vi "TwoCameraDisplayPanel.vi"() -> ()   [LabVIEW 2013]
uses:
  MvLVLib/MvCameraControl.lvlib
  MvLVLib/VIs/CreateGigEHandle.vi
  MvLVLib/VIs/CreateU3VHandle.vi
  <vilib>/picture/picture.llb/imagedata.ctl
panel:
  out "GenTLDeviceArray":T1(array[cluster])
  in  "image data 2":T2 caption="图像数据"
  in  "Rectangle 2":T3
  out "pFrameInfoEx out 2":T4
  in  "pConvertInfo In 2":T5
  out "nWidth 2":u32
  out "nHeight 2":u32
  out "PayloadSize 2":u32
  out "PixelFormat 2":u32
  out "handle out 2":u64
  in  "handle 2":u64
  out "Picture 2":picture
  in  "Device List 2":u16(ring)
  out "U3VDeviceArray":T6(array[cluster])
  out "GigEDeviceArray":T7(array[cluster])
  in  "pConvertInfo In":T5
  out "PixelFormat":u32
  out "handle out":u64
  in  "handle":u64
  in  "Rectangle":T3
  in  "image data":T2 caption="图像数据"
  out "Picture":picture
  out "PayloadSize":u32
  out "pFrameInfoEx out":T4
  out "nHeight":u32
  out "nWidth":u32
  out "Acquisision Flag":bool
  in  "Trigger Mode":bool
  in  "Continuous":bool
  out "打开标志":bool
  in  "stop":bool
  in  "Trigger Once":bool
  in  "Stop":bool
  in  "Start":bool
  in  "Open Device":bool
  in  "Close Device":bool
  in  "error in (no error) 2":errorcluster caption="错误输入（无错误）"
  in  "Refresh Devices":bool
  in  "Device List":u16(ring)
  # "Initialize"
  # "Acquisition"
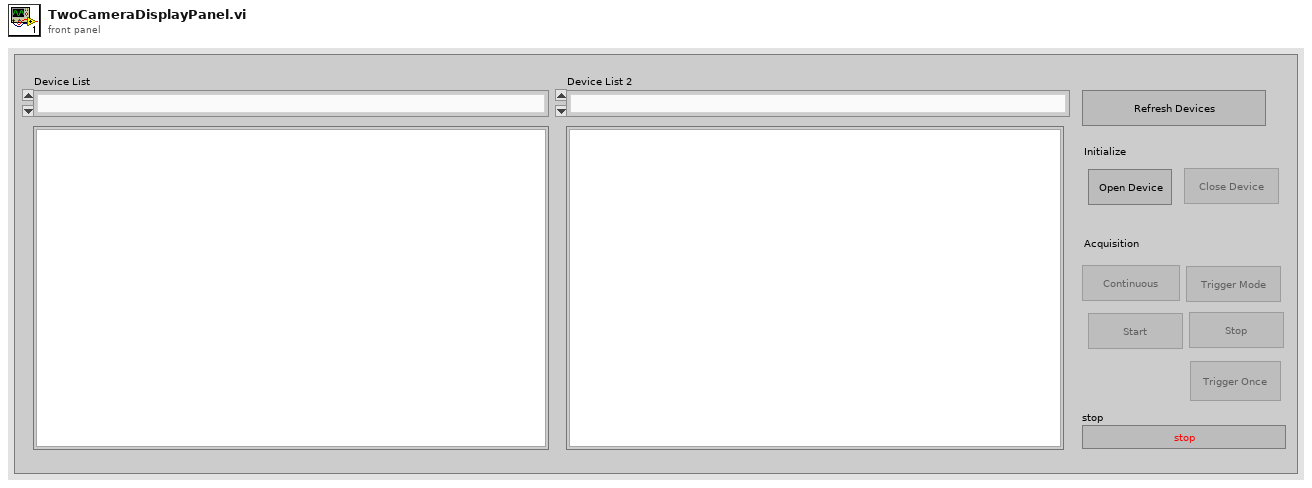
[diagram p1: front panel]
types:
  T1 = cluster{"nMajorVer":u16, "nMinorVer":u16, "nMacAddrHigh":u32, "nMacAddrLow":u32, "nTLayerType":u32, "nReserved0":u32, "nReserved1":u32, "nReserved2":u32, "nReserved3":u32, "chInterfaceID":string, "chVendorName":string, "chModelName":string, "chManufacturerInfo":string, "chDeviceVersion":string, "chSerialNumber":string, "chUserDefinedName":string, "chDeviceID":string, "nRes0":u32, "nRes1":u32, "nRes2":u32, "nRes3":u32, "nRes4":u32, "nRes5":u32, "nRes6":u32}[]
  T2 = typedef "imagedata.ctl" = cluster{"image type":i32, "image depth":i32, "image":u8[], "mask":u8[], "colors":u32[], "Rectangle":cluster{"left":i16, "top":i16, "right":i16, "bottom":i16}}
  T3 = cluster{"left":i16, "top":i16, "right":i16, "bottom":i16}
  T4 = cluster{"nWidth":u16, "nHeight":u16, "enPixelType":i32, "nFrameNum":u32, "nDevTimeStampHigh":u32, "nDevTimeStampLow":u32, "nReserved0":u32, "nHostTimeStamp":i64, "nFrameLen":u32, "nSecondCount]":u32, "nCycleCount":u32, "nCycleOffset":u32, "fGain":u32, "fExposureTime":u32, "nAverageBrightness":u32, "nRed":u32, "nGreen":u32, "nBlue":u32, "nFrameCounter":u32, "nTriggerIndex":u32, "nInput":u32, "nOutput":u32, "nOffsetX":u32, "nOffsetY":u32, "nReserved[0]":u32, "nReserved[1]":u32, "nReserved[2]":u32, "nReserved[3]":u32, "nReserved[4]":u32, "nReserved[5]":u32, "nReserved[6]":u32, "nReserved[7]":u32, "nReserved[8]":u32, "nReserved[9]":u32, "nReserved[10]":u32, "nReserved[11]":u32, "nReserved[12]":u32, "nReserved[13]":u32, "nReserved[14] 10":u32, "nReserved[15] 11":u32, "nReserved[16] 12":u32, "nReserved[17] 13":u32, "nReserved[18] 14":u32, "nReserved[19] 15":u32, "nReserved[20] 16":u32, "nReserved[21] 17":u32, "nReserved[22] 18":u32, "nReserved[23] 19":u32, "nReserved[24] 20":u32, "nReserved[25] 21":u32, "nReserved[26] 22":u32, "nReserved[27] 23":u32, "nReserved[28] 24":u32, "nReserved[29] 25":u32, "nReserved[30] 26":u32, "nReserved[31] 27":u32, "nReserved[32] 28":u32, "nReserved[33] 29":u32, "nReserved[34] 30":u32, "nReserved[35] 31":u32, "nReserved[36] 32":u32, "nReserved[37] 33":u32, "nReserved[38] 34":u32, "nReserved[39] 35":u32, "nReserved[40] 36":u32}
  T5 = cluster{"nWidth":u16, "nHeight":u16, "enSrcPixelType":u32, "nSrcDataLen":u32, "enDstPixelType":u32, "nDstLen":u32, "nDstBufferSize":u32, "nRes0":u32, "nRes1":u32, "nRes2":u32, "nRes3":u32}
  T6 = cluster{"nMajorVer":u16, "nMinorVer":u16, "nMacAddrHigh":u32, "nMacAddrLow":u32, "nTLayerType":u32, "nReserved0":u32, "nReserved1":u32, "nReserved2":u32, "nReserved3":u32, "CrtlInEndPoint":u8, "CrtlOutEndPoint":u8, "StreamEndPoint":u8, "EventEndPoint":u8, "idVendor":u16, "idProduct":u16, "nDeviceNumber":u32, "chDeviceGUID":string, "chVendorName":string, "chModelName":string, "chFamilyName":string, "chDeviceVersion":string, "chManufacturerName":string, "chSerialNumber":string, "chUserDefinedName":string, "nbcdUSB":u32, "nDeviceAddress":u32, "nRes0":u32, "nRes1":u32, "nResAlign":u32}[]
  T7 = cluster{"nMajorVer":u16, "nMinorVer":u16, "nMacAddrHigh":u32, "nMacAddrLow":u32, "nTLayerType":u32, "nReserved0":u32, "nReserved1":u32, "nReserved2":u32, "nReserved3":u32, "nIpCfgOption":u32, "nIpCfgCurrent":u32, "nCurrentIp":u32, "nCurrentSubNetMask":u32, "nDefaultGateWay":u32, "chManualfacturerName":string, "chModelName":string, "chDeviceVersion":string, "chManufacturerSpecificInfo":string, "chSerialNumber":string, "chUserDefinedName":string, "nNetExport":u32, "nRes0":u32, "nRes1":u32, "nRes2":u32, "nRes3":u32}[]
  T8 = enum8{"Enabled", "Disabled", "Disabled and Grayed Out"}
  T9 = cluster{"nCurValue":u32, "nMax":u32, "nMin":u32, "nInc":u32, "nReserved[0]":u32, "nReserved[1]":u32, "nReserved[2]":u32, "nReserved[3]":u32}
  T10 = cluster{"nCurValue":u32, "nSupportedNum":u32, "nSupportValue":u32[], "nReserved[0]":u32, "nReserved[1]":u32, "nReserved[2]":u32, "nReserved[3]":u32}
  T11 = cluster{"nMajorVer":u16, "nMinorVer":u16, "nMacAddrHigh":u32, "nMacAddrLow":u32, "nTLayerType":u32, "nReserved0":u32, "nReserved1":u32, "nReserved2":u32, "nReserved3":u32, "nIpCfgOption":u32, "nIpCfgCurrent":u32, "nCurrentIp":u32, "nCurrentSubNetMask":u32, "nDefaultGateWay":u32, "chManualfacturerName":string, "chModelName":string, "chDeviceVersion":string, "chManufacturerSpecificInfo":string, "chSerialNumber":string, "chUserDefinedName":string, "nNetExport":u32, "nRes0":u32, "nRes1":u32, "nRes2":u32, "nRes3":u32}
  T12 = cluster{"nMajorVer":u16, "nMinorVer":u16, "nMacAddrHigh":u32, "nMacAddrLow":u32, "nTLayerType":u32, "nReserved0":u32, "nReserved1":u32, "nReserved2":u32, "nReserved3":u32, "CrtlInEndPoint":u8, "CrtlOutEndPoint":u8, "StreamEndPoint":u8, "EventEndPoint":u8, "idVendor":u16, "idProduct":u16, "nDeviceNumber":u32, "chDeviceGUID":string, "chVendorName":string, "chModelName":string, "chFamilyName":string, "chDeviceVersion":string, "chManufacturerName":string, "chSerialNumber":string, "chUserDefinedName":string, "nbcdUSB":u32, "nDeviceAddress":u32, "nRes0":u32, "nRes1":u32, "nResAlign":u32}
  T13 = cluster{"nMajorVer":u16, "nMinorVer":u16, "nMacAddrHigh":u32, "nMacAddrLow":u32, "nTLayerType":u32, "nReserved0":u32, "nReserved1":u32, "nReserved2":u32, "nReserved3":u32, "chInterfaceID":string, "chVendorName":string, "chModelName":string, "chManufacturerInfo":string, "chDeviceVersion":string, "chSerialNumber":string, "chUserDefinedName":string, "chDeviceID":string, "nRes0":u32, "nRes1":u32, "nRes2":u32, "nRes3":u32, "nRes4":u32, "nRes5":u32, "nRes6":u32}
  T14 = cluster{"nWidth":u32, "nHeight":u32, "enSrcPixelType":u32, "nSrcDataLen":u32, "enDstPixelType":u32, "nDstLen":u32, "nDstBufferSize":u32, "nRes0":u32, "nRes1":u32, "nRes2":u32, "nRes3":u32}
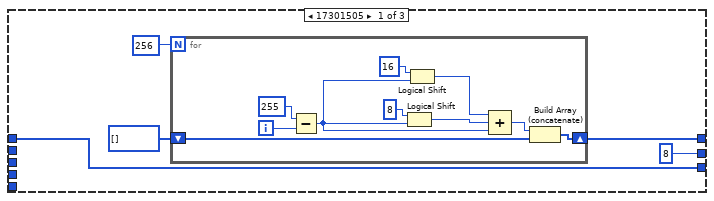
[diagram p9: hidden frame]
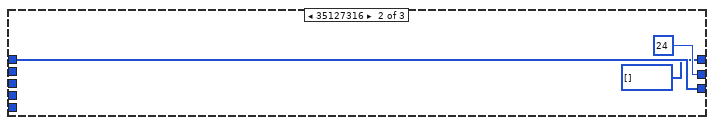
[diagram p10: hidden frame]
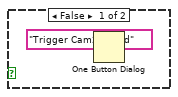
[diagram p12: hidden frame]
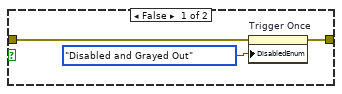
[diagram p17: hidden frame]
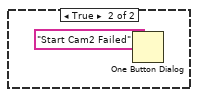
[diagram p18: hidden frame]
diagram:
  n1 = while {
    tunnel: ["stop"] -> w3
    shift-right: [w41] -> _
    shift-left: "handle" -> [_]
    tunnel: ["stop"] -> w1
    tunnel: [w10] -> _
    stop <- "stop" stop-if-true
    n2 = property on="handle out" class="DigNum (strict)"() -> ("Value"=w33:u64)  [unwired: 2 in, 2 out]
    n3 = property on="handle out" class="DigNum (strict)"() -> ("Value"=w39:u64)  [unwired: 2 in, 2 out]
    n4 = property on="handle out" class="DigNum (strict)"() -> ("Value"=w34:u64)  [unwired: 2 in, 2 out]
    n5 = property on="handle out" class="DigNum (strict)"() -> ("Value"=w35:u64)  [unwired: 2 in, 2 out]
    n6 = property on="handle out 2" class="DigNum (strict)"() -> ("Value"=w24:u64)  [unwired: 2 in, 2 out]
    n7 = property on="handle out" class="DigNum (strict)"() -> ("Value"=w38:u64)  [unwired: 2 in, 2 out]
    n8 = property on="handle out" class="DigNum (strict)"() -> ("Value"=w37:u64)  [unwired: 2 in, 2 out]
    n9 = property on="handle out 2" class="DigNum (strict)"() -> ("Value"=w18:u64)  [unwired: 2 in, 2 out]
    n10 = property on="handle out 2" class="DigNum (strict)"() -> ("Value"=w17:u64)  [unwired: 2 in, 2 out]
    n11 = case shown="True" "Trigger Mode" {
      tunnel: w34 -> [_ w401]
      frame False {
      }
      frame True {
        n12 = call "SetEnumValue.vi"("nValue"=u32 1, "strKey"="TriggerMode", "handle"=w401) -> ("error out"=w407:errorcluster)  [unwired: 6 in, 2 out]
        n13 = call "SetEnumValue.vi"("error in (no error)"=w407, "nValue"=u32 7, "strKey"="TriggerSource", "handle"=w401) -> ("error out"=w406:errorcluster)  [unwired: 5 in, 2 out]
        n14 = property on="Trigger Mode" class="Bool"(error in=w406, "DisabledEnum"=T8."Disabled and Grayed Out" ("禁用")) -> (error out=w405:errorcluster)  [unwired: 1 in, 1 out]
        n15 = property on="Continuous" class="Bool"(error in=w405, "DisabledEnum"=T8."Enabled" ("禁用")) -> (error out=w403:errorcluster)  [unwired: 1 in, 1 out]
        n16 = property on="Trigger Once" class="Bool"(error in=w403, "DisabledEnum"=T8."Enabled" ("禁用")) -> ()  [unwired: 1 in, 2 out]
      }
    }
    n17 = case shown="True" "Trigger Once" {
      tunnel: w38 -> [_ w416]
      frame False {
      }
      frame True {
        n18 = call "SetCommandValue.vi"("strValue"="TriggerSoftware", "handle"=w416) -> ("function return"=w414:i32)  [unwired: 7 in, 2 out]
        n19 = Equal To 0?(x=w414) -> (x = 0?=w413:bool)
        n20 = case shown="True" w413 {
          frame False {
            n21 = One Button Dialog(message="Trigger Cam1 Failed") -> ()  [unwired: 1 in, 1 out]
          }
          frame True {
            n22 = One Button Dialog(message="Trigger Can1 Success") -> ()  [unwired: 1 in, 1 out]
          }
        }
      }
    }
    n23 = case shown="True" "Stop" {
      tunnel: w37 -> [_ w391]
      frame False {
      }
      frame True {
        n24 = call "StopGrabbing.vi"("handle"=w391) -> ("error out"=w390:errorcluster)  [unwired: 8 in, 2 out]
        n25 = property on="Acquisision Flag" class="Bool (strict)"(error in=w390, "Value"=FALSE ("采集标志")) -> (error out=w385:errorcluster)  [unwired: 1 in, 1 out]
        n26 = property on="Start" class="Bool"(error in=w385, "DisabledEnum"=T8."Enabled" ("禁用")) -> (error out=w384:errorcluster)  [unwired: 1 in, 1 out]
        n27 = property on="Stop" class="Bool"(error in=w384, "DisabledEnum"=T8."Disabled and Grayed Out" ("禁用")) -> (error out=w383:errorcluster)  [unwired: 1 in, 1 out]
        n28 = property on="Trigger Once" class="Bool"(error in=w383, "DisabledEnum"=T8."Disabled and Grayed Out" ("禁用")) -> ()  [unwired: 1 in, 2 out]
      }
    }
    n29 = case shown="True" "Continuous" {
      tunnel: w33 -> [_ w392]
      frame False {
      }
      frame True {
        n30 = call "SetEnumValue.vi"("nValue"=u32 0, "strKey"="TriggerMode", "handle"=w392) -> ("error out"=w393:errorcluster)  [unwired: 6 in, 2 out]
        n31 = property on="Continuous" class="Bool"(error in=w393, "DisabledEnum"=T8."Disabled and Grayed Out" ("禁用")) -> (error out=w397:errorcluster)  [unwired: 1 in, 1 out]
        n32 = property on="Trigger Mode" class="Bool"(error in=w397, "DisabledEnum"=T8."Enabled" ("禁用")) -> (error out=w395:errorcluster)  [unwired: 1 in, 1 out]
        n33 = property on="Trigger Once" class="Bool"(error in=w395, "DisabledEnum"=T8."Disabled and Grayed Out" ("禁用")) -> ()  [unwired: 1 in, 2 out]
      }
    }
    n34 = case shown="True" "Stop" {
      tunnel: w18 -> [_ w147]
      frame False {
      }
      frame True {
        n35 = call "StopGrabbing.vi"("handle"=w147) -> ("error out"=w146:errorcluster)  [unwired: 8 in, 2 out]
        n36 = property on="Acquisision Flag" class="Bool (strict)"(error in=w146, "Value"=FALSE ("采集标志")) -> (error out=w141:errorcluster)  [unwired: 1 in, 1 out]
        n37 = property on="Start" class="Bool"(error in=w141, "DisabledEnum"=T8."Enabled" ("禁用")) -> (error out=w140:errorcluster)  [unwired: 1 in, 1 out]
        n38 = property on="Stop" class="Bool"(error in=w140, "DisabledEnum"=T8."Disabled and Grayed Out" ("禁用")) -> (error out=w139:errorcluster)  [unwired: 1 in, 1 out]
        n39 = property on="Trigger Once" class="Bool"(error in=w139, "DisabledEnum"=T8."Disabled and Grayed Out" ("禁用")) -> ()  [unwired: 1 in, 2 out]
      }
    }
    n40 = case shown="True" "Trigger Once" {
      tunnel: w17 -> [_ w136]
      frame False {
      }
      frame True {
        n41 = call "SetCommandValue.vi"("strValue"="TriggerSoftware", "handle"=w136) -> ("function return"=w134:i32)  [unwired: 7 in, 2 out]
        n42 = Equal To 0?(x=w134) -> (x = 0?=w133:bool)
        n43 = case shown="True" w133 {
          frame False {
            n44 = One Button Dialog(message="Trigger Cam2 Failed") -> ()  [unwired: 1 in, 1 out]
          }
          frame True {
            n45 = One Button Dialog(message="Trigger Cam2 Success") -> ()  [unwired: 1 in, 1 out]
          }
        }
      }
    }
    n46 = case shown="True" "Close Device" {
      tunnel: w39 -> [_ w462]
      frame False {
      }
      frame True {
        n47 = call "CloseDevice.vi"("handle"=w462) -> ("error out"=w464:errorcluster, "handle out"=w461:u64)  [unwired: 8 in, 1 out]
        n48 = call "DestroyHandle.vi"("error in (no error)"=w464, "handle"=w461) -> ("error out"=w463:errorcluster)  [unwired: 8 in, 1 out]
        n49 = property on="Open Device" class="Bool"(error in=w463, "DisabledEnum"=T8."Enabled" ("禁用")) -> (error out=w477:errorcluster)  [unwired: 1 in, 1 out]
        n50 = property on="Close Device" class="Bool"(error in=w477, "DisabledEnum"=T8."Disabled and Grayed Out" ("禁用")) -> (error out=w476:errorcluster)  [unwired: 1 in, 1 out]
        n51 = property on="Start" class="Bool"(error in=w476, "DisabledEnum"=T8."Disabled and Grayed Out" ("禁用")) -> (error out=w475:errorcluster)  [unwired: 1 in, 1 out]
        n52 = property on="Stop" class="Bool"(error in=w475, "DisabledEnum"=T8."Disabled and Grayed Out" ("禁用")) -> (error out=w474:errorcluster)  [unwired: 1 in, 1 out]
        n53 = property on="Trigger Once" class="Bool"(error in=w474, "DisabledEnum"=T8."Disabled and Grayed Out" ("禁用")) -> (error out=w471:errorcluster)  [unwired: 1 in, 1 out]
        n54 = property on="Continuous" class="Bool"(error in=w471, "DisabledEnum"=T8."Disabled and Grayed Out" ("禁用")) -> (error out=w469:errorcluster)  [unwired: 1 in, 1 out]
        n55 = property on="Trigger Mode" class="Bool"(error in=w469, "DisabledEnum"=T8."Disabled and Grayed Out" ("禁用")) -> (error out=w468:errorcluster)  [unwired: 1 in, 1 out]
        n56 = property on="打开标志" class="Bool (strict)"(error in=w468, "Value"=FALSE ("打开标志")) -> (error out=w466:errorcluster)  [unwired: 1 in, 1 out]
        n57 = property on="Acquisision Flag" class="Bool (strict)"(error in=w466, "Value"=FALSE ("采集标志")) -> ()  [unwired: 1 in, 2 out]
      }
    }
    n58 = case shown="True" "Refresh Devices" {
      tunnel: [w547 w556] -> w29
      tunnel: "error in (no error) 2" -> [w547 w555]
      frame False {
        n59 = property on="GigEDeviceArray" class="Arr (strict)" props=["Value"]() -> ()  [unwired: 2 in, 3 out]
        n60 = property on="U3VDeviceArray" class="Arr (strict)" props=["Value"]() -> ()  [unwired: 2 in, 3 out]
      }
      frame True {
        n61 = call "EnumDevicesEx2.vi"("nLayerType"=u32 965, "error in (no error)"=w555) -> ("GigEDeviceArray"=w552:T7, "U3VDeviceArray"=w550:T6, "GenTLDevice"=w549:T1, "error out"=w556:errorcluster)  [unwired: 8 in, 2 out]
        "GigEDeviceArray" <- w552
        "U3VDeviceArray" <- w550
        "GenTLDeviceArray" <- w549
        n62 = for {
          tunnel: w556 -> [_]
          tunnel: w552 -> [w583] mode=indexing
          tunnel: [w582] -> w554 mode=indexing
          n63 = Unbundle By Name(w583) -> ("chUserDefinedName"=w586:string)
          n64 = Unbundle By Name(w583) -> ("chSerialNumber"=w584:string)
          n65 = Unbundle By Name(w583) -> ("chModelName"=w585:string)
          n66 = call <vilib>:"Space Constant.vi"() -> ("String"=w589:string)
          n67 = Concatenate Strings("[GigE] " ("字符串"), w586, w589, w585, "(" ("字符串"), w584, ")" ("字符串")) -> (w582:string)
        }
        n68 = for {
          tunnel: w550 -> [w576] mode=indexing
          tunnel: [w573] -> w553 mode=indexing
          n69 = Unbundle By Name(w576) -> ("chUserDefinedName"=w580:string)
          n70 = Unbundle By Name(w576) -> ("chSerialNumber"=w575:string)
          n71 = Unbundle By Name(w576) -> ("chModelName"=w578:string)
          n72 = call <vilib>:"Space Constant.vi"() -> ("String"=w579:string)
          n73 = Concatenate Strings("[U3V] " ("字符串"), w580, w579, w578, "(" ("字符串"), w575, ")" ("字符串")) -> (w573:string)
        }
        n74 = for {
          tunnel: w549 -> [w564] mode=indexing
          tunnel: [w562] -> w548 mode=indexing
          n75 = Unbundle By Name(w564) -> ("nTLayerType"=w559:u32, "chUserDefinedName"=w567:string, "chModelName"=w561:string, "chSerialNumber"=w560:string)
          n76 = case shown="80" w559 {
            tunnel: ["[GenTL]" ("字符串") "[GenTL CML]" ("字符串") "[GenTL CXP]" ("字符串") "[GenTL XOF]" ("字符串")] -> w558
            frame Default {
            }
            frame 128 {
            }
            frame 256 {
            }
            frame 512 {
            }
          }
          n77 = call <vilib>:"Space Constant.vi"() -> ("String"=w566:string)
          n78 = Concatenate Strings(w558, w567, w566, w561, "(" ("字符串"), w560, ")" ("字符串")) -> (w562:string)
        }
        n79 = Build Array (concatenate)(w554, w553, w548) -> (w551:string[])
        n80 = property on="Device List" class="Ring (strict)"("Strings []"=w551) -> ()  [unwired: 2 in, 2 out]
        n81 = property on="Device List 2" class="Ring (strict)"("Strings []"=w551) -> ()  [unwired: 2 in, 2 out]
      }
    }
    n82 = case shown="True" "Start" {
      tunnel: w35 -> [_ w423]
      frame False {
      }
      frame True {
        n83 = call "GetIntValue.vi"("strKey"="PayloadSize", "handle"=w423) -> ("error out"=w429:errorcluster, "pIntValue out"=w425:T9, "handle out"=w421:u64)  [unwired: 6 in, 1 out]
        n84 = Unbundle By Name(w425) -> ("nCurValue"=→"PayloadSize":u32)
        n85 = call "GetEnumValue.vi"("error in (no error)"=w429, "strKey"="PixelFormat", "handle"=w421) -> ("error out"=w428:errorcluster, "pEnumValue out"=w430:T10, "handle out"=w420:u64)  [unwired: 5 in, 1 out]
        n86 = Unbundle By Name(w430) -> ("nCurValue"=→"PixelFormat":u32)
        n87 = call "StartGrabbing.vi"("error in (no error)"=w428, "handle"=w420) -> ("error out"=w427:errorcluster, "function return"=w433:i32, "handle out"=w419:u64)  [unwired: 7 in]
        n88 = Not Equal To 0?(x=w433) -> (x != 0?=w432:bool)
        n89 = case shown="True" w432 {
          tunnel: w423 -> [_ _]
          tunnel: w427 -> [w436 _]
          tunnel: w419 -> [w435 _]
          frame False {
            n90 = call "GetIntValue.vi"("error in (no error)"=w436, "strKey"="Width", "handle"=w435) -> ("error out"=w443:errorcluster, "pIntValue out"=w437:T9, "handle out"=w434:u64)  [unwired: 5 in, 1 out]
            n91 = Unbundle By Name(w437) -> ("nCurValue"=→"nWidth":u32)
            n92 = call "GetIntValue.vi"("error in (no error)"=w443, "strKey"="Height", "handle"=w434) -> ("error out"=w442:errorcluster, "pIntValue out"=w440:T9)  [unwired: 5 in, 2 out]
            n93 = Unbundle By Name(w440) -> ("nCurValue"=→"nHeight":u32)
            n94 = property on="Start" class="Bool"(error in=w442, "DisabledEnum"=T8."Disabled and Grayed Out" ("禁用")) -> (error out=w452:errorcluster)  [unwired: 1 in, 1 out]
            n95 = property on="Stop" class="Bool"(error in=w452, "DisabledEnum"=T8."Enabled" ("禁用")) -> (error out=w438:errorcluster)  [unwired: 1 in, 1 out]
            n96 = property on="Continuous" class="Bool"(error in=w438) -> (error out=w448:errorcluster, "DisabledEnum"=w449:T8)  [unwired: 1 in, 1 out]
            n97 = Equal To 0?(x=w449) -> (x = 0?=w450:bool)
            n98 = case shown="True" w450 {
              tunnel: w448 -> [w455 w458]
              tunnel: [w454 w457] -> w447
              frame False {
                n99 = property on="Trigger Once" class="Bool"(error in=w455, "DisabledEnum"=T8."Disabled and Grayed Out" ("禁用")) -> (error out=w454:errorcluster)  [unwired: 1 in, 1 out]
              }
              frame True {
                n100 = property on="Trigger Once" class="Bool"(error in=w458, "DisabledEnum"=T8."Enabled" ("禁用")) -> (error out=w457:errorcluster)  [unwired: 1 in, 1 out]
              }
            }
            n101 = property on="Acquisision Flag" class="Bool (strict)"(error in=w447, "Value"=TRUE ("采集标志")) -> ()  [unwired: 1 in, 2 out]
          }
          frame True {
            n102 = One Button Dialog(message="Start Cam1 Failed") -> ()  [unwired: 1 in, 1 out]
          }
        }
      }
    }
    n103 = case shown="True" "Start" {
      tunnel: w24 -> [_ w171]
      frame False {
      }
      frame True {
        n104 = call "GetIntValue.vi"("strKey"="PayloadSize", "handle"=w171) -> ("error out"=w177:errorcluster, "pIntValue out"=w173:T9, "handle out"=w169:u64)  [unwired: 6 in, 1 out]
        n105 = Unbundle By Name(w173) -> ("nCurValue"=→"PayloadSize 2":u32)
        n106 = call "GetEnumValue.vi"("error in (no error)"=w177, "strKey"="PixelFormat", "handle"=w169) -> ("error out"=w176:errorcluster, "pEnumValue out"=w178:T10, "handle out"=w168:u64)  [unwired: 5 in, 1 out]
        n107 = Unbundle By Name(w178) -> ("nCurValue"=→"PixelFormat 2":u32)
        n108 = call "StartGrabbing.vi"("error in (no error)"=w176, "handle"=w168) -> ("error out"=w175:errorcluster, "function return"=w181:i32, "handle out"=w167:u64)  [unwired: 7 in]
        n109 = Not Equal To 0?(x=w181) -> (x != 0?=w180:bool)
        n110 = case shown="False" w180 {
          tunnel: w171 -> [_ _]
          tunnel: w175 -> [w186 _]
          tunnel: w167 -> [w185 _]
          frame False {
            n111 = call "GetIntValue.vi"("error in (no error)"=w186, "strKey"="Width", "handle"=w185) -> ("error out"=w192:errorcluster, "pIntValue out"=w187:T9, "handle out"=w184:u64)  [unwired: 5 in, 1 out]
            n112 = Unbundle By Name(w187) -> ("nCurValue"=→"nWidth 2":u32)
            n113 = call "GetIntValue.vi"("error in (no error)"=w192, "strKey"="Height", "handle"=w184) -> ("error out"=w183:errorcluster, "pIntValue out"=w190:T9)  [unwired: 5 in, 2 out]
            n114 = Unbundle By Name(w190) -> ("nCurValue"=→"nHeight 2":u32)
            n115 = property on="Start" class="Bool"(error in=w183, "DisabledEnum"=T8."Disabled and Grayed Out" ("禁用")) -> ()  [unwired: 1 in, 2 out]
            n116 = property on="Stop" class="Bool"("DisabledEnum"=T8."Enabled" ("禁用")) -> (error out=w188:errorcluster)  [unwired: 2 in, 1 out]
            n117 = property on="Continuous" class="Bool"(error in=w188) -> (error out=w197:errorcluster, "DisabledEnum"=w198:T8)  [unwired: 1 in, 1 out]
            n118 = Equal To 0?(x=w198) -> (x = 0?=w199:bool)
            n119 = case shown="True" w199 {
              tunnel: w197 -> [w202 w205]
              tunnel: [w201 w204] -> w196
              frame False {
                n120 = property on="Trigger Once" class="Bool"(error in=w202, "DisabledEnum"=T8."Disabled and Grayed Out" ("禁用")) -> (error out=w201:errorcluster)  [unwired: 1 in, 1 out]
              }
              frame True {
                n121 = property on="Trigger Once" class="Bool"(error in=w205, "DisabledEnum"=T8."Enabled" ("禁用")) -> (error out=w204:errorcluster)  [unwired: 1 in, 1 out]
              }
            }
            n122 = property on="Acquisision Flag" class="Bool (strict)"(error in=w196, "Value"=TRUE ("采集标志")) -> ()  [unwired: 1 in, 2 out]
          }
          frame True {
            n123 = One Button Dialog(message="Start Cam2 Failed") -> ()  [unwired: 1 in, 1 out]
          }
        }
      }
    }
    n124 = property on="PayloadSize" class="DigNum (strict)"() -> ("Value"=w30:u32)  [unwired: 2 in, 2 out]
    n125 = property on="PayloadSize 2" class="DigNum (strict)"() -> ("Value"=w12:u32)  [unwired: 2 in, 2 out]
    n126 = property on="handle out" class="DigNum (strict)"() -> ("Value"=w36:u64)  [unwired: 2 in, 2 out]
    n127 = property on="Acquisision Flag" class="Bool (strict)"() -> ("Value"=w8:bool)  [unwired: 2 in, 2 out]
    n128 = property on="Acquisision Flag" class="Bool (strict)"() -> ("Value"=w9:bool)  [unwired: 2 in, 2 out]
    n129 = Initialize Array(u8 0 ("元素"), w30) -> (w31:u8[])
    n130 = property on="handle out 2" class="DigNum (strict)"() -> ("Value"=w15:u64)  [unwired: 2 in, 2 out]
    n131 = Initialize Array(u8 0 ("元素"), w12) -> (w13:u8[])
    n132 = property on="handle out 2" class="DigNum (strict)"() -> ("Value"=w20:u64)  [unwired: 2 in, 2 out]
    n133 = property on="handle out 2" class="DigNum (strict)"() -> ("Value"=w22:u64)  [unwired: 2 in, 2 out]
    n134 = property on="handle" class="DigNum (strict)"() -> ("Value"=w40:u64)  [unwired: 2 in, 2 out]
    n135 = case shown="True" "Open Device" {
      tunnel: [w482 w495] -> _
      tunnel: w40 -> [w482 w484]
      tunnel: w29 -> [_ w490]
      frame False {
      }
      frame True {
        n136 = property on="handle out" class="DigNum (strict)"() -> ("Value"=w492:u64)  [unwired: 2 in, 2 out]
        n137 = property on="Device List" class="Ring (strict)"() -> ("RingText.Text"=w488:string)  [unwired: 2 in, 2 out]
        n138 = call "DestroyHandle.vi"("error in (no error)"=w490, "handle"=w492) -> ("error out"=w491:errorcluster)  [unwired: 8 in, 1 out]
        n139 = call <vilib>:"Clear Errors.vi"("error in (no error)"=w491) -> ("error out"=w483:errorcluster)  [unwired: 5 in, 1 out]
        n140 = String Subset(string=w488, length (rest)=5 ("长度（剩余）")) -> (substring=w487:string)  [unwired: 1 in]
        n141 = case shown="\"[GenT\"" w487 {
          tunnel: [w504 w510 w522 w525] -> w486
          tunnel: [w503 w509 w521 w526] -> w485
          tunnel: w484 -> [_ _ _ w526]
          tunnel: w483 -> [_ _ _ w525]
          frame "[GigE" {
            n142 = local read "GigEDeviceArray"() -> (w502:T7)
            n143 = property on="Device List" class="Ring (strict)"() -> ("Value"=w505:u16)  [unwired: 2 in, 2 out]
            n144 = Index Array(array=w502, index=w505) -> (element=w501:T11)
            n145 = call-poly "CreateHandle.vi"("GigEDevice"=w501) -> ("error out"=w504:errorcluster, "handle"=w503:u64)  [unwired: 7 in, 1 out]
          }
          frame "[U3V]" {
            n146 = local read "GigEDeviceArray"() -> (w507:T7)
            n147 = property on="Device List" class="Ring (strict)"() -> ("Value"=w513:u16)  [unwired: 2 in, 2 out]
            n148 = local read "U3VDeviceArray"() -> (w508:T6)
            n149 = Array Size(array=w507) -> (size(s)=w512:i32)
            n150 = Subtract(x=w513, y=w512) -> (x-y=w511:i32)
            n151 = Index Array(array=w508, index=w511) -> (element=w506:T12)
            n152 = call-poly "CreateHandle.vi"("U3VDevice"=w506) -> ("error out"=w510:errorcluster, "handle"=w509:u64)  [unwired: 7 in, 1 out]
          }
          frame "[GenT" {
            n153 = local read "GigEDeviceArray"() -> (w515:T7)
            n154 = local read "U3VDeviceArray"() -> (w514:T6)
            n155 = property on="Device List" class="Ring (strict)"() -> ("Value"=w524:u16)  [unwired: 2 in, 2 out]
            n156 = Array Size(array=w515) -> (size(s)=w523:i32)
            n157 = local read "GenTLDeviceArray"() -> (w520:T1)
            n158 = Subtract(x=w524, y=w523) -> (x-y=w519:i32)
            n159 = Array Size(array=w514) -> (size(s)=w518:i32)
            n160 = Subtract(x=w519, y=w518) -> (x-y=w517:i32)
            n161 = Index Array(array=w520, index=w517) -> (element=w516:T13)
            n162 = call "CreateCMLHandle.vi"("GenTLCMLDevice"=w516) -> ("error out"=w522:errorcluster, "handle"=w521:u64)  [unwired: 7 in, 1 out]
          }
          frame Default {
          }
        }
        "handle out" <- w485
        n163 = call "OpenDevice.vi"("error in (no error)"=w486, "nSwitchoverKey"=u16 0, "nAccessMode"=u32 1, "handle"=w485) -> ("error out"=w496:errorcluster, "return"=w494:i32, "handle out"=w493:u64)  [unwired: 5 in]
        n164 = Not Equal?(x=w494, y=0) -> (x != y?=w499:bool)
        n165 = case shown="True" w499 {
          tunnel: w493 -> [w527 w544]
          tunnel: w496 -> [w528 _]
          tunnel: [w527 u64 0 ("handle")] -> w495
          frame False {
            n166 = call "SetEnumValue.vi"("error in (no error)"=w528, "nValue"=u32 0, "strKey"="TriggerMode", "handle"=w527) -> ("error out"=w539:errorcluster)  [unwired: 5 in, 2 out]
            n167 = property on="Start" class="Bool"(error in=w539, "DisabledEnum"=T8."Enabled" ("禁用")) -> (error out=w537:errorcluster)  [unwired: 1 in, 1 out]
            n168 = property on="Open Device" class="Bool"(error in=w537, "DisabledEnum"=T8."Disabled and Grayed Out" ("禁用")) -> (error out=w536:errorcluster)  [unwired: 1 in, 1 out]
            n169 = property on="Close Device" class="Bool"(error in=w536, "DisabledEnum"=T8."Enabled" ("禁用")) -> (error out=w533:errorcluster)  [unwired: 1 in, 1 out]
            n170 = property on="Trigger Mode" class="Bool"(error in=w533, "DisabledEnum"=T8."Enabled" ("禁用")) -> (error out=w531:errorcluster)  [unwired: 1 in, 1 out]
            n171 = property on="Continuous" class="Bool"(error in=w531, "DisabledEnum"=T8."Disabled and Grayed Out" ("禁用")) -> (error out=w529:errorcluster)  [unwired: 1 in, 1 out]
            n172 = property on="打开标志" class="Bool (strict)"(error in=w529, "Value"=TRUE ("布尔")) -> ()  [unwired: 1 in, 2 out]
          }
          frame True {
            n173 = call "DestroyHandle.vi"("handle"=w544) -> ()  [unwired: 9 in, 2 out]
            n174 = property on="打开标志" class="Bool (strict)"("Value"=FALSE) -> ()  [unwired: 2 in, 2 out]
            n175 = One Button Dialog(message="Open Cam1 Failed") -> ()  [unwired: 1 in, 1 out]
          }
        }
      }
    }
    n176 = property on="PayloadSize 2" class="DigNum (strict)"() -> ("Value"=w6:u32)  [unwired: 2 in, 2 out]
    n177 = Initialize Array(u8 0 ("元素"), w6) -> (w4:u8[])
    n178 = property on="handle 2" class="DigNum (strict)"() -> ("Value"=w28:u64)  [unwired: 2 in, 2 out]
    n179 = case shown="True" w9 {
      tunnel: w36 -> [_ w302]
      tunnel: w31 -> [_ w301]
      tunnel: w30 -> [_ w300]
      frame False {
      }
      frame True {
        n180 = property on="PayloadSize" class="DigNum (strict)"() -> ("Value"=w296:u32)  [unwired: 2 in, 2 out]
        n181 = call "GetOneFrameTimeout.vi"("handle"=w302, "pData"=w301, "nDataSize"=w300, "nMsec"=1000) -> ("function return"=w299:i32, "pData Out"=w298:u8[], "pFrameInfoEx out"=w297:T4)  [unwired: 7 in, 2 out]
        n182 = Equal To 0?(x=w299) -> (x = 0?=w304:bool)
        n183 = Initialize Array(u8 0 ("元素"), w296) -> (w294:u8[])
        n184 = case shown="True" w304 {
          tunnel: w298 -> [_ w316]
          tunnel: w297 -> [_ w319]
          tunnel: w294 -> [_ w314]
          frame False {
          }
          frame True {
            w329 = i16 0 ("left")
            n185 = Unbundle By Name(w319) -> ("nWidth"=w311:u16, "nHeight"=w313:u16, "enPixelType"=w306:i32, "nFrameLen"=w315:u32)
            n186 = Compound Arithmetic op=AND(w306, -2147483648 ("value")) -> (w317:i32)
            n187 = case shown="80000000" w317 {
              tunnel: w314 -> [_ w347]
              tunnel: w316 -> [w337 w346]
              tunnel: w315 -> [w334 w345]
              tunnel: [w337 w342] -> w312
              tunnel: [w336 w341] -> w310
              tunnel: [w335 w340] -> w309
              tunnel: [w333 w339] -> w308
              tunnel: [w334 w338] -> w307
              tunnel: w311 -> [w336 _]
              tunnel: w313 -> [w335 _]
              tunnel: w306 -> [w333 _]
              frame Default {
              }
              frame -2147483648 {
                # "HB格式"
                n188 = property on="PayloadSize" class="DigNum (strict)"() -> ("Value"=w344:u32)  [unwired: 2 in, 2 out]
                n189 = property on="handle out" class="DigNum (strict)"() -> ("Value"=w348:u64)  [unwired: 2 in, 2 out]
                n190 = call "HBDecode.vi"("handle"=w348, "pSrcData"=w346, "pDstBuf In"=w347, "SrcDataLen"=w345, "DstBufferSize"=w344) -> ("pDstBuf Out"=w342:u8[], "pHBDecode Out"=w343:T14)  [unwired: 6 in, 3 out]
                n191 = Unbundle By Name(w343) -> ("nWidth"=w341:u32, "nHeight"=w340:u32, "enDstPixelType"=w339:u32, "nDstLen"=w338:u32)
              }
            }
            n192 = property on="Picture" class="Pict"() -> ("Width"=w324:u32)  [unwired: 2 in, 2 out]
            n193 = Divide(x=w324, y=w310) -> (x/y=w323:dbl)
            n194 = case shown="Default" w308 {
              selector: w308 -> [_ _ w369]
              tunnel: w312 -> [w351 w366 w379]
              tunnel: w309 -> [_ _ w367]
              tunnel: w310 -> [_ _ w370]
              tunnel: [w351 w366 w371] -> w322
              tunnel: [8 24 24] -> w320
              tunnel: [w349 i32[] [] i32[] []] -> w321
              tunnel: w307 -> [_ _ w368]
              frame 17301505 {
                n195 = for {
                  N: 256 -> [_]
                  shift-right: [w358] -> w349
                  shift-left: i32[] [] ("数组") -> [w357]
                  i -> [w354]
                  n196 = Subtract(x=255, y=w354) -> (x-y=w355:i32)
                  n197 = Logical Shift(y=i16 8, x=w355) -> (x << y=w360:i32)
                  n198 = Logical Shift(y=16 ("x"), x=w355) -> (x << y=w361:i32)
                  n199 = Compound Arithmetic op=ADD(w361, w360, w355) -> (w359:i32)
                  n200 = Build Array (concatenate)(w359, w357) -> (w358:i32[])
                }
              }
              frame 35127316 {
              }
              frame Default {
                n201 = Compound Arithmetic op=MULTIPLY(w367, w370, u32 3 ("值")) -> (w375:u32)
                n202 = Bundle By Name(cluster="pConvertInfo In", "nWidth"=w370, "nHeight"=w367, "enSrcPixelType"=w369, "nSrcDataLen"=w368, "enDstPixelType"=u32 35127316, "nDstBufferSize"=w375) -> (w374:T5)
                n203 = property on="handle out" class="DigNum (strict)"() -> ("Value"=w380:u64)  [unwired: 2 in, 2 out]
                n204 = Initialize Array(u8 0 ("元素"), w375) -> (w378:u8[])
                n205 = call "ConvertPixelType.vi"("handle"=w380, "pSrcData"=w379, "pDstBuf In"=w378, "pConvertInfo In"=w374) -> ("pDstBuf Out"=w371:u8[])  [unwired: 7 in, 4 out]
              }
            }
            n206 = property on="Picture" class="Pict"("ZoomFactor"=w323) -> ()  [unwired: 2 in, 2 out]
            n207 = Bundle By Name(cluster="Rectangle", "left"=w329, "top"=w329, "right"=w310, "bottom"=w309) -> (w326:T3)
            n208 = Bundle By Name(cluster="image data", "image type"=0, "image depth"=w320, "image"=w322, "mask"=u8[] [], "colors"=w321, "Rectangle"=w326) -> (w325:T2)
            n209 = call <vilib>:"Draw Flattened Pixmap.vi"("image data"=w325) -> ("new picture"=→"Picture":picture)  [unwired: 8 in]
            "pFrameInfoEx out" <- w319
          }
        }
        n210 = Wait (ms)(milliseconds to wait=u32 10 ("等待时间（毫秒）")) -> ()  [unwired: 1 out]
      }
    }
    n211 = case shown="True" w8 {
      tunnel: w15 -> [_ w50]
      tunnel: w13 -> [_ w49]
      tunnel: w12 -> [_ w48]
      tunnel: w4 -> [_ w44]
      frame False {
      }
      frame True {
        n212 = call "GetOneFrameTimeout.vi"("handle"=w50, "pData"=w49, "nDataSize"=w48, "nMsec"=1000) -> ("function return"=w47:i32, "pData Out"=w46:u8[], "pFrameInfoEx out"=w45:T4)  [unwired: 7 in, 2 out]
        n213 = Equal To 0?(x=w47) -> (x = 0?=w52:bool)
        n214 = case shown="True" w52 {
          tunnel: w46 -> [_ w63]
          tunnel: w45 -> [_ w67]
          tunnel: w44 -> [_ w64]
          frame False {
          }
          frame True {
            w80 = i16 0 ("left")
            n215 = Unbundle By Name(w67) -> ("nWidth"=w62:u16, "nHeight"=w61:u16, "enPixelType"=w54:i32, "nFrameLen"=w60:u32)
            n216 = Compound Arithmetic op=AND(w54, -2147483648 ("value")) -> (w65:i32)
            n217 = case shown="80000000" w65 {
              tunnel: [w85 w93] -> w55
              tunnel: [w84 w92] -> w57
              tunnel: [w83 w91] -> w56
              tunnel: [w81 w90] -> w59
              tunnel: [w82 w89] -> w58
              tunnel: w64 -> [_ w88]
              tunnel: w63 -> [w85 w87]
              tunnel: w60 -> [_ w86]
              tunnel: w62 -> [w84 _]
              tunnel: w61 -> [w83 _]
              tunnel: w60 -> [w82 _]
              tunnel: w54 -> [w81 _]
              frame Default {
              }
              frame -2147483648 {
                # "HB格式"
                n218 = property on="PayloadSize 2" class="DigNum (strict)"() -> ("Value"=w95:u32)  [unwired: 2 in, 2 out]
                n219 = property on="handle out 2" class="DigNum (strict)"() -> ("Value"=w96:u64)  [unwired: 2 in, 2 out]
                n220 = call "HBDecode.vi"("handle"=w96, "pSrcData"=w87, "pDstBuf In"=w88, "SrcDataLen"=w86, "DstBufferSize"=w95) -> ("pDstBuf Out"=w93:u8[], "pHBDecode Out"=w94:T14)  [unwired: 6 in, 3 out]
                n221 = Unbundle By Name(w94) -> ("nWidth"=w92:u32, "nHeight"=w91:u32, "enDstPixelType"=w90:u32, "nDstLen"=w89:u32)
              }
            }
            n222 = case shown="Default" w54 {
              tunnel: w55 -> [w99 w114 w129]
              tunnel: w56 -> [_ _ w126]
              tunnel: w57 -> [_ _ w125]
              tunnel: [w99 w114 w119] -> w73
              tunnel: [8 24 24] -> w68
              tunnel: [w97 i32[] [] i32[] []] -> w72
              tunnel: w57 -> [_ _ w118]
              tunnel: w56 -> [_ _ w117]
              tunnel: w59 -> [_ _ w116]
              tunnel: w58 -> [_ _ w115]
              frame 17301505 {
                n223 = for {
                  N: 256 -> [_]
                  shift-right: [w106] -> w97
                  shift-left: i32[] [] ("数组") -> [w105]
                  i -> [w102]
                  n224 = Subtract(x=255, y=w102) -> (x-y=w103:i32)
                  n225 = Logical Shift(y=i16 8, x=w103) -> (x << y=w108:i32)
                  n226 = Logical Shift(y=16 ("x"), x=w103) -> (x << y=w109:i32)
                  n227 = Compound Arithmetic op=ADD(w109, w108, w103) -> (w107:i32)
                  n228 = Build Array (concatenate)(w107, w105) -> (w106:i32[])
                }
              }
              frame 35127316 {
              }
              frame Default {
                n229 = Compound Arithmetic op=MULTIPLY(w126, w125, u32 3 ("值")) -> (w123:u32)
                n230 = Bundle By Name(cluster="pConvertInfo In 2", "nWidth"=w118, "nHeight"=w117, "enSrcPixelType"=w116, "nSrcDataLen"=w115, "enDstPixelType"=u32 35127316, "nDstBufferSize"=w123) -> (w122:T5)
                n231 = property on="handle out 2" class="DigNum (strict)"() -> ("Value"=w130:u64)  [unwired: 2 in, 2 out]
                n232 = Initialize Array(u8 0 ("元素"), w123) -> (w128:u8[])
                n233 = call "ConvertPixelType.vi"("handle"=w130, "pSrcData"=w129, "pDstBuf In"=w128, "pConvertInfo In"=w122) -> ("pDstBuf Out"=w119:u8[])  [unwired: 7 in, 4 out]
              }
            }
            n234 = property on="Picture 2" class="Pict"() -> ("Width"=w75:u32)  [unwired: 2 in, 2 out]
            n235 = Divide(x=w75, y=w57) -> (x/y=w74:dbl)
            n236 = property on="Picture 2" class="Pict"("ZoomFactor"=w74) -> ()  [unwired: 2 in, 2 out]
            n237 = Bundle By Name(cluster="Rectangle 2", "left"=w80, "top"=w80, "right"=w57, "bottom"=w56) -> (w77:T3)
            n238 = Bundle By Name(cluster="image data 2", "image type"=0, "image depth"=w68, "image"=w73, "mask"=u8[] [], "colors"=w72, "Rectangle"=w77) -> (w76:T2)
            n239 = call <vilib>:"Draw Flattened Pixmap.vi"("image data"=w76) -> ("new picture"=→"Picture 2":picture)  [unwired: 8 in]
            "pFrameInfoEx out 2" <- w67
          }
        }
        n240 = Wait (ms)(milliseconds to wait=u32 10 ("等待时间（毫秒）")) -> ()  [unwired: 1 out]
      }
    }
    n241 = case shown="True" "Trigger Mode" {
      tunnel: w22 -> [_ w158]
      frame False {
      }
      frame True {
        n242 = call "SetEnumValue.vi"("nValue"=u32 1, "strKey"="TriggerMode", "handle"=w158) -> ("error out"=w162:errorcluster)  [unwired: 6 in, 2 out]
        n243 = call "SetEnumValue.vi"("error in (no error)"=w162, "nValue"=u32 7, "strKey"="TriggerSource", "handle"=w158) -> ("error out"=w157:errorcluster)  [unwired: 5 in, 2 out]
        n244 = property on="Trigger Mode" class="Bool"(error in=w157, "DisabledEnum"=T8."Disabled and Grayed Out" ("禁用")) -> ()  [unwired: 1 in, 2 out]
        n245 = property on="Continuous" class="Bool"("DisabledEnum"=T8."Enabled" ("禁用")) -> (error out=w160:errorcluster)  [unwired: 2 in, 1 out]
        n246 = property on="Trigger Once" class="Bool"(error in=w160, "DisabledEnum"=T8."Enabled" ("禁用")) -> ()  [unwired: 1 in, 2 out]
      }
    }
    n247 = case shown="True" "Continuous" {
      tunnel: w20 -> [_ w150]
      frame False {
      }
      frame True {
        n248 = call "SetEnumValue.vi"("nValue"=u32 0, "strKey"="TriggerMode", "handle"=w150) -> ("error out"=w149:errorcluster)  [unwired: 6 in, 2 out]
        n249 = property on="Continuous" class="Bool"(error in=w149, "DisabledEnum"=T8."Disabled and Grayed Out" ("禁用")) -> ()  [unwired: 1 in, 2 out]
        n250 = property on="Trigger Mode" class="Bool"("DisabledEnum"=T8."Enabled" ("禁用")) -> (error out=w152:errorcluster)  [unwired: 2 in, 1 out]
        n251 = property on="Trigger Once" class="Bool"(error in=w152, "DisabledEnum"=T8."Disabled and Grayed Out" ("禁用")) -> ()  [unwired: 1 in, 2 out]
      }
    }
    n252 = case shown="True" "Open Device" {
      tunnel: [w229 w242] -> _
      tunnel: w28 -> [w229 w230]
      tunnel: w29 -> [_ w237]
      frame False {
      }
      frame True {
        n253 = property on="handle out 2" class="DigNum (strict)"() -> ("Value"=w238:u64)  [unwired: 2 in, 2 out]
        n254 = property on="Device List 2" class="Ring (strict)"() -> ("RingText.Text"=w235:string)  [unwired: 2 in, 2 out]
        n255 = call "DestroyHandle.vi"("error in (no error)"=w237, "handle"=w238) -> ("error out"=w239:errorcluster)  [unwired: 8 in, 1 out]
        n256 = call <vilib>:"Clear Errors.vi"("error in (no error)"=w239) -> ("error out"=w231:errorcluster)  [unwired: 5 in, 1 out]
        n257 = String Subset(string=w235, length (rest)=5 ("长度（剩余）")) -> (substring=w234:string)  [unwired: 1 in]
        n258 = case shown="Default" w234 {
          tunnel: [w251 w257 w269 w273] -> w232
          tunnel: [w250 w256 w268 w272] -> w233
          tunnel: w231 -> [_ _ _ w273]
          tunnel: w230 -> [_ _ _ w272]
          frame "[GigE" {
            n259 = local read "GigEDeviceArray"() -> (w249:T7)
            n260 = property on="Device List 2" class="Ring (strict)"() -> ("Value"=w252:u16)  [unwired: 2 in, 2 out]
            n261 = Index Array(array=w249, index=w252) -> (element=w248:T11)
            n262 = call-poly "CreateHandle.vi"("GigEDevice"=w248) -> ("error out"=w251:errorcluster, "handle"=w250:u64)  [unwired: 7 in, 1 out]
          }
          frame "[U3V]" {
            n263 = local read "GigEDeviceArray"() -> (w254:T7)
            n264 = property on="Device List 2" class="Ring (strict)"() -> ("Value"=w260:u16)  [unwired: 2 in, 2 out]
            n265 = local read "U3VDeviceArray"() -> (w255:T6)
            n266 = Array Size(array=w254) -> (size(s)=w259:i32)
            n267 = Subtract(x=w260, y=w259) -> (x-y=w258:i32)
            n268 = Index Array(array=w255, index=w258) -> (element=w253:T12)
            n269 = call-poly "CreateHandle.vi"("U3VDevice"=w253) -> ("error out"=w257:errorcluster, "handle"=w256:u64)  [unwired: 7 in, 1 out]
          }
          frame "[GenT" {
            n270 = local read "GigEDeviceArray"() -> (w262:T7)
            n271 = local read "U3VDeviceArray"() -> (w261:T6)
            n272 = property on="Device List 2" class="Ring (strict)"() -> ("Value"=w271:u16)  [unwired: 2 in, 2 out]
            n273 = Array Size(array=w262) -> (size(s)=w270:i32)
            n274 = local read "GenTLDeviceArray"() -> (w267:T1)
            n275 = Subtract(x=w271, y=w270) -> (x-y=w266:i32)
            n276 = Array Size(array=w261) -> (size(s)=w265:i32)
            n277 = Subtract(x=w266, y=w265) -> (x-y=w264:i32)
            n278 = Index Array(array=w267, index=w264) -> (element=w263:T13)
            n279 = call "CreateCMLHandle.vi"("GenTLCMLDevice"=w263) -> ("error out"=w269:errorcluster, "handle"=w268:u64)  [unwired: 7 in, 1 out]
          }
          frame Default {
          }
        }
        "handle out 2" <- w233
        n280 = call "OpenDevice.vi"("error in (no error)"=w232, "nSwitchoverKey"=u16 0, "nAccessMode"=u32 1, "handle"=w233) -> ("error out"=w243:errorcluster, "return"=w241:i32, "handle out"=w240:u64)  [unwired: 5 in]
        n281 = Not Equal?(x=w241, y=0) -> (x != y?=w246:bool)
        n282 = case shown="False" w246 {
          tunnel: w240 -> [w274 w291]
          tunnel: w243 -> [w275 _]
          tunnel: [w274 u64 0 ("handle")] -> w242
          frame False {
            n283 = call "SetEnumValue.vi"("error in (no error)"=w275, "nValue"=u32 0, "strKey"="TriggerMode", "handle"=w274) -> ("error out"=w286:errorcluster)  [unwired: 5 in, 2 out]
            n284 = property on="Start" class="Bool"(error in=w286, "DisabledEnum"=T8."Enabled" ("禁用")) -> (error out=w284:errorcluster)  [unwired: 1 in, 1 out]
            n285 = property on="Open Device" class="Bool"(error in=w284, "DisabledEnum"=T8."Disabled and Grayed Out" ("禁用")) -> (error out=w283:errorcluster)  [unwired: 1 in, 1 out]
            n286 = property on="Close Device" class="Bool"(error in=w283, "DisabledEnum"=T8."Enabled" ("禁用")) -> (error out=w280:errorcluster)  [unwired: 1 in, 1 out]
            n287 = property on="Trigger Mode" class="Bool"(error in=w280, "DisabledEnum"=T8."Enabled" ("禁用")) -> (error out=w278:errorcluster)  [unwired: 1 in, 1 out]
            n288 = property on="Continuous" class="Bool"(error in=w278, "DisabledEnum"=T8."Disabled and Grayed Out" ("禁用")) -> (error out=w276:errorcluster)  [unwired: 1 in, 1 out]
            n289 = property on="打开标志" class="Bool (strict)"(error in=w276, "Value"=TRUE ("布尔")) -> ()  [unwired: 1 in, 2 out]
          }
          frame True {
            n290 = call "DestroyHandle.vi"("handle"=w291) -> ()  [unwired: 9 in, 2 out]
            n291 = property on="打开标志" class="Bool (strict)"("Value"=FALSE) -> ()  [unwired: 2 in, 2 out]
            n292 = One Button Dialog(message="Open Cam2 Failed") -> ()  [unwired: 1 in, 1 out]
          }
        }
      }
    }
    n293 = property on="handle out 2" class="DigNum (strict)"() -> ("Value"=w26:u64)  [unwired: 2 in, 2 out]
    n294 = case shown="True" "Close Device" {
      tunnel: w26 -> [_ w208]
      frame False {
      }
      frame True {
        n295 = call "CloseDevice.vi"("handle"=w208) -> ("error out"=w211:errorcluster, "handle out"=w209:u64)  [unwired: 8 in, 1 out]
        n296 = call "DestroyHandle.vi"("error in (no error)"=w211, "handle"=w209) -> ("error out"=w210:errorcluster)  [unwired: 8 in, 1 out]
        n297 = property on="Open Device" class="Bool"(error in=w210, "DisabledEnum"=T8."Enabled" ("禁用")) -> (error out=w224:errorcluster)  [unwired: 1 in, 1 out]
        n298 = property on="Close Device" class="Bool"(error in=w224, "DisabledEnum"=T8."Disabled and Grayed Out" ("禁用")) -> (error out=w223:errorcluster)  [unwired: 1 in, 1 out]
        n299 = property on="Start" class="Bool"(error in=w223, "DisabledEnum"=T8."Disabled and Grayed Out" ("禁用")) -> (error out=w222:errorcluster)  [unwired: 1 in, 1 out]
        n300 = property on="Stop" class="Bool"(error in=w222, "DisabledEnum"=T8."Disabled and Grayed Out" ("禁用")) -> (error out=w221:errorcluster)  [unwired: 1 in, 1 out]
        n301 = property on="Trigger Once" class="Bool"(error in=w221, "DisabledEnum"=T8."Disabled and Grayed Out" ("禁用")) -> (error out=w218:errorcluster)  [unwired: 1 in, 1 out]
        n302 = property on="Continuous" class="Bool"(error in=w218, "DisabledEnum"=T8."Disabled and Grayed Out" ("禁用")) -> (error out=w216:errorcluster)  [unwired: 1 in, 1 out]
        n303 = property on="Trigger Mode" class="Bool"(error in=w216, "DisabledEnum"=T8."Disabled and Grayed Out" ("禁用")) -> (error out=w215:errorcluster)  [unwired: 1 in, 1 out]
        n304 = property on="打开标志" class="Bool (strict)"(error in=w215, "Value"=FALSE ("打开标志")) -> (error out=w213:errorcluster)  [unwired: 1 in, 1 out]
        n305 = property on="Acquisision Flag" class="Bool (strict)"(error in=w213, "Value"=FALSE ("采集标志")) -> ()  [unwired: 1 in, 2 out]
      }
    }
    n306 = property on="handle out 2" class="DigNum (strict)"() -> ("Value"=w10:u64)  [unwired: 2 in, 2 out]
    n307 = property on="handle out" class="DigNum (strict)"() -> ("Value"=w41:u64)  [unwired: 2 in, 2 out]
  }
  n308 = flat-sequence {
    tunnel: w3 -> [w593]
    tunnel: w1 -> [w590]
    frame #0 {
      n309 = property on="handle out" class="DigNum (strict)"() -> ("Value"=w592:u64)  [unwired: 2 in, 2 out]
      n310 = case shown="True" w593 {
        tunnel: w592 -> [_ w629]
        frame False {
        }
        frame True {
          n311 = property on="打开标志" class="Bool (strict)"() -> ("Value"=w620:bool)  [unwired: 2 in, 2 out]
          n312 = case shown="True" w620 {
            tunnel: w629 -> [_ w636]
            frame False {
            }
            frame True {
              n313 = call "CloseDevice.vi"("handle"=w636) -> ("error out"=w637:errorcluster, "handle out"=w635:u64)  [unwired: 8 in, 1 out]
              n314 = call "DestroyHandle.vi"("error in (no error)"=w637, "handle"=w635) -> ()  [unwired: 8 in, 2 out]
            }
          }
          n315 = property on="Open Device" class="Bool"("DisabledEnum"=T8."Enabled" ("禁用")) -> (error out=w628:errorcluster)  [unwired: 2 in, 1 out]
          n316 = property on="Close Device" class="Bool"(error in=w628, "DisabledEnum"=T8."Disabled and Grayed Out" ("禁用")) -> (error out=w627:errorcluster)  [unwired: 1 in, 1 out]
          n317 = property on="Trigger Once" class="Bool"(error in=w627, "DisabledEnum"=T8."Disabled and Grayed Out" ("禁用")) -> (error out=w626:errorcluster)  [unwired: 1 in, 1 out]
          n318 = property on="Start" class="Bool"(error in=w626, "DisabledEnum"=T8."Disabled and Grayed Out" ("禁用")) -> (error out=w625:errorcluster)  [unwired: 1 in, 1 out]
          n319 = property on="Stop" class="Bool"(error in=w625, "DisabledEnum"=T8."Disabled and Grayed Out" ("禁用")) -> (error out=w624:errorcluster)  [unwired: 1 in, 1 out]
          n320 = property on="Continuous" class="Bool"(error in=w624, "DisabledEnum"=T8."Disabled and Grayed Out" ("禁用")) -> (error out=w622:errorcluster)  [unwired: 1 in, 1 out]
          n321 = property on="Trigger Mode" class="Bool"(error in=w622, "DisabledEnum"=T8."Disabled and Grayed Out" ("禁用")) -> (error out=w617:errorcluster)  [unwired: 1 in, 1 out]
          n322 = property on="打开标志" class="Bool (strict)"(error in=w617, "Value"=FALSE ("打开标志")) -> (error out=w616:errorcluster)  [unwired: 1 in, 1 out]
          n323 = property on="Acquisision Flag" class="Bool (strict)"(error in=w616, "Value"=FALSE ("采集标志")) -> ()  [unwired: 1 in, 2 out]
        }
      }
      n324 = property on="handle out 2" class="DigNum (strict)"() -> ("Value"=w591:u64)  [unwired: 2 in, 2 out]
      n325 = case shown="True" w590 {
        tunnel: w591 -> [_ w607]
        frame False {
        }
        frame True {
          n326 = property on="打开标志" class="Bool (strict)"() -> ("Value"=w598:bool)  [unwired: 2 in, 2 out]
          n327 = case shown="True" w598 {
            tunnel: w607 -> [_ w614]
            frame False {
            }
            frame True {
              n328 = call "CloseDevice.vi"("handle"=w614) -> ("error out"=w615:errorcluster, "handle out"=w613:u64)  [unwired: 8 in, 1 out]
              n329 = call "DestroyHandle.vi"("error in (no error)"=w615, "handle"=w613) -> ()  [unwired: 8 in, 2 out]
            }
          }
          n330 = property on="Open Device" class="Bool"("DisabledEnum"=T8."Enabled" ("禁用")) -> (error out=w606:errorcluster)  [unwired: 2 in, 1 out]
          n331 = property on="Close Device" class="Bool"(error in=w606, "DisabledEnum"=T8."Disabled and Grayed Out" ("禁用")) -> (error out=w605:errorcluster)  [unwired: 1 in, 1 out]
          n332 = property on="Trigger Once" class="Bool"(error in=w605, "DisabledEnum"=T8."Disabled and Grayed Out" ("禁用")) -> (error out=w604:errorcluster)  [unwired: 1 in, 1 out]
          n333 = property on="Start" class="Bool"(error in=w604, "DisabledEnum"=T8."Disabled and Grayed Out" ("禁用")) -> (error out=w603:errorcluster)  [unwired: 1 in, 1 out]
          n334 = property on="Stop" class="Bool"(error in=w603, "DisabledEnum"=T8."Disabled and Grayed Out" ("禁用")) -> (error out=w602:errorcluster)  [unwired: 1 in, 1 out]
          n335 = property on="Continuous" class="Bool"(error in=w602, "DisabledEnum"=T8."Disabled and Grayed Out" ("禁用")) -> (error out=w600:errorcluster)  [unwired: 1 in, 1 out]
          n336 = property on="Trigger Mode" class="Bool"(error in=w600, "DisabledEnum"=T8."Disabled and Grayed Out" ("禁用")) -> (error out=w595:errorcluster)  [unwired: 1 in, 1 out]
          n337 = property on="打开标志" class="Bool (strict)"(error in=w595, "Value"=FALSE ("打开标志")) -> (error out=w594:errorcluster)  [unwired: 1 in, 1 out]
          n338 = property on="Acquisision Flag" class="Bool (strict)"(error in=w594, "Value"=FALSE ("采集标志")) -> ()  [unwired: 1 in, 2 out]
        }
      }
    }
    frame #1 {
      n339 = call "Finalize.vi"() -> ()  [unwired: 10 in, 2 out]
    }
  }
